vi "ErrorToVolts.vi"(1 "Reading":dbl, 2 "UI Data":T1) -> (0 "Voltage":dbl)   [LabVIEW 2014]
uses:
  controls/UI Data.ctl
  controls/BridgeSettings.ctl
  Driver/Typedefs/OutputChannelTypedef.ctl
  controls/ChannelSelection.ctl
  Driver/Typedefs/InputChannelTypedef.ctl
  Driver/YbTempCtrl.lvlib
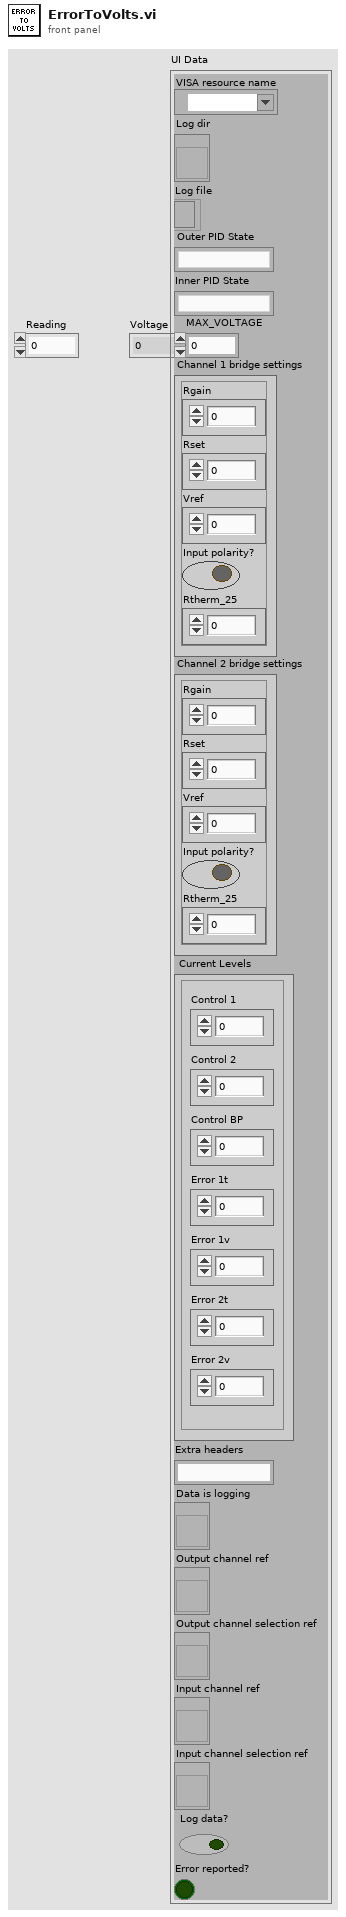
[diagram p1: front panel]
types:
  T1 = typedef "UI Data.ctl" = cluster{"VISA resource name":refnum<visa-resource-name>, "Log dir":refnum<vi>, "Log file":refnum<file>, "Outer PID State":string, "Inner PID State":string, "MAX_VOLTAGE":dbl, "Channel 1 bridge settings":T2, "Channel 2 bridge settings":T2, "Current Levels":cluster{"Control 1":dbl, "Control 2":dbl, "Control BP":dbl, "Error 1t":dbl, "Error 1v":dbl, "Error 2t":dbl, "Error 2v":dbl}, "Extra headers":string, "Data is logging":refnum<vi>, "Output channel ref":refnum<vi>, "Output channel selection ref":refnum<vi>, "Input channel ref":refnum<vi>, "Input channel selection ref":refnum<vi>, "Log data?":bool, "Error reported?":bool}
  T2 = typedef "BridgeSettings.ctl" = cluster{"Rgain":dbl, "Rset":dbl, "Vref":dbl, "Input polarity?":bool, "Rtherm_25":dbl}
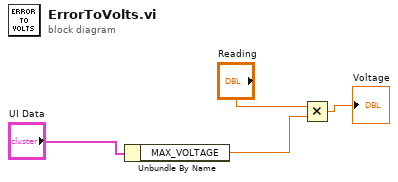
[diagram p0: block diagram]
diagram:
  n1 = Unbundle By Name("UI Data") -> ("MAX_VOLTAGE"=w1:dbl)
  n2 = Multiply(x="Reading", y=w1) -> (x*y=→"Voltage":dbl)
